vi "WSVCAP SHL Host TL Tester.vi"() -> ()   [LabVIEW 2012]
uses:
  Type Defs/WSVCAP SHL DUT Number Enum.ctl
  <vilib>/userdefined/High Color/nirio_resource_hc.ctl
  Type Defs/WSVCAP SHL Tester System Cluster.ctl
  Type Defs/WSVCAP SHL I2C DUT Mask Mode Enum.ctl
panel:
  in  "Mode":enum32{"C1", "C2", "C3", "All", "Single"}(radio)
  in  "RFFE Slave Address":u8=144 caption="Slave Address" format="0x%02x"
  in  "RFFE Mode":enum32{"Write/Read", "Cycle"}(tab)
  in  "Read Data DUT":string caption="Read Data Out"
  in  "Read DUT":bool
  in  "Enable DUT":bool
  in  "Disable DUT":bool
  in  "Write DUT":bool
  in  "Write Data DUT":string caption="Write Data Out"
  out "Read Data DUT":string caption="Data In"
  out "Cycle Count":u64=2 min=1 max=4 step=1 format="%#.4p"
  in  "Number of Commands":u32=2 min=1 max=4 step=1
  in  "Post Command Delay":dbl[](array[numeric])=[5e-06, 5e-06] min=0.0 max=0.5 format="%#.0p s"
  in  "Command":string[](array[string])=["4200000000", "421F7F1F7F"]
  in  "Start RFFE Cycle":bool
  in  "Stop RFFE Cycle":bool
  out "Activity Log":string
  out "Simulate FPGA":bool
  out "Online":bool
  out "FPGA Resource":T1
  out "Status":string
  out "Busy":bool
  in  "I2C Bytes to Read":u8=1 caption="Bytes" min=1 max=4 step=1
  in  "Device":enum32{"C1", "C2", "C3"}(radio)
  in  "Exit":bool
  out "Read Data I2C":u8[](array[numeric]) caption="Data In" format="0x%02x"
  in  "Read Reg I2C":u8 caption="Register" format="0x%02x"
  in  "Read I2C":bool
  in  "DUT":T2
  in  "Write Data I2C":u8 caption="Data Out" format="0x%02x"
  in  "Write Reg I2C":u8=144 caption="Register" format="0x%02x"
  in  "I2C Init":bool
  in  "Init Data":u8[](array[numeric])=[164, 160, 14, 33] caption="Data Out" format="0x%02x"
  in  "Init Reg":u8[](array[numeric])=[191, 7, 9, 10] caption="Register" format="0x%02x"
  in  "Write I2C":bool
  in  "Monitor":bool
  in  "I2C Slave Address":u8=144 caption="Slave Address" format="0x%02x"
  out "AD7747 Values":string[][](table)
  in  "RFFE Clock Rate (Hz)":dbl=1000000.0 caption="Clock Rate" format="%.1p Hz"
  in  "I2C Clock Rate (Hz)":dbl=100000.0 caption="Clock Rate" format="%.0p Hz"
  in  "Error":errorcluster
  # "WS1050 Tester"
  # "AD7747 (I2C)"
  # "DUT (RFFE)"
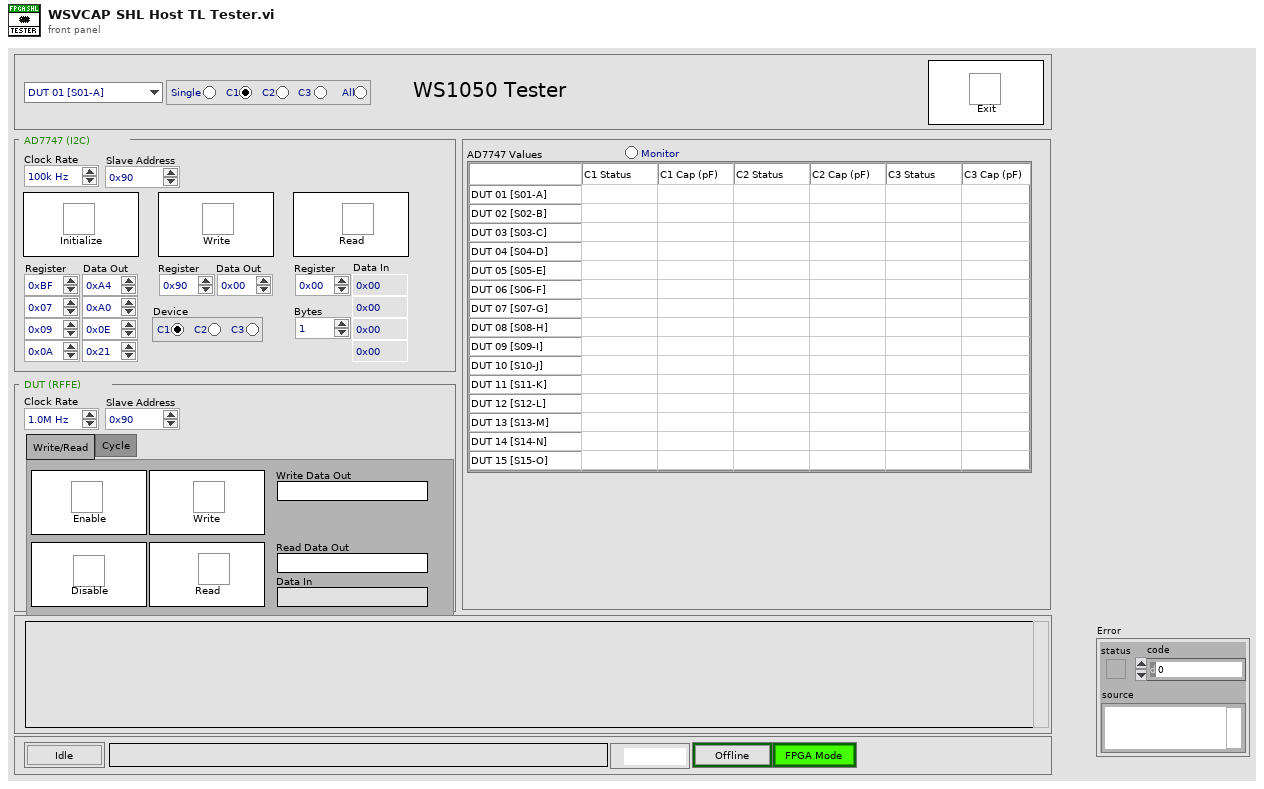
[diagram p1: front panel]
types:
  T1 = typedef "nirio_resource_hc.ctl" = tag
  T2 = typedef "WSVCAP SHL DUT Number Enum.ctl" = enum16{"DUT 01 [S01-A]", "DUT 02 [S02-B]", "DUT 03 [S03-C]", "DUT 04 [S04-D]", "DUT 05 [S05-E]", "DUT 06 [S06-F]", "DUT 07 [S07-G]", "DUT 08 [S08-H]", "DUT 09 [S09-I]", "DUT 10 [S10-J]", "DUT 11 [S11-K]", "DUT 12 [S12-L]", "DUT 13 [S13-M]", "DUT 14 [S14-N]", "DUT 15 [S15-O]", "DUT 16 [S16-P]"}
  T3 = typedef "WSVCAP SHL Tester System Cluster.ctl" = cluster{"I2C Monitor":bool, "SPI Cyle":bool, "SPI Mode":enum32{"Write/Read", "Cycle"}, "RFFE Cyle":bool, "RFFE Mode":enum32{"Write/Read", "Cycle"}}
  T4 = enum8{"Enabled", "Disabled", "Disabled and Grayed Out"}
  T5 = typedef "WSVCAP SHL I2C DUT Mask Mode Enum.ctl" = enum16{"Custom", "C1", "C2", "C3", "All"}
  T6 = typedef "WSVCAP SHL Core System Cluster.ctl" = cluster{"Settings":T7, "FPGA Resource":tag, "Online":bool, "I2C Wait Ticks":u32, "SPI Wait Ticks":u32, "RFFE Wait Ticks":u32}
  T7 = typedef "WSVCAP SHL I2C Settings Cluster.ctl" = cluster{"FPGA Resource Name":string, "I2C Slave Address":u8, "I2C Clock Rate (Hz)":dbl, "SPI Clock Rate (Hz)":dbl, "RFFE Slave Address":u8, "RFFE Clock Rate (Hz)":dbl, "Simulate FPGA":bool}
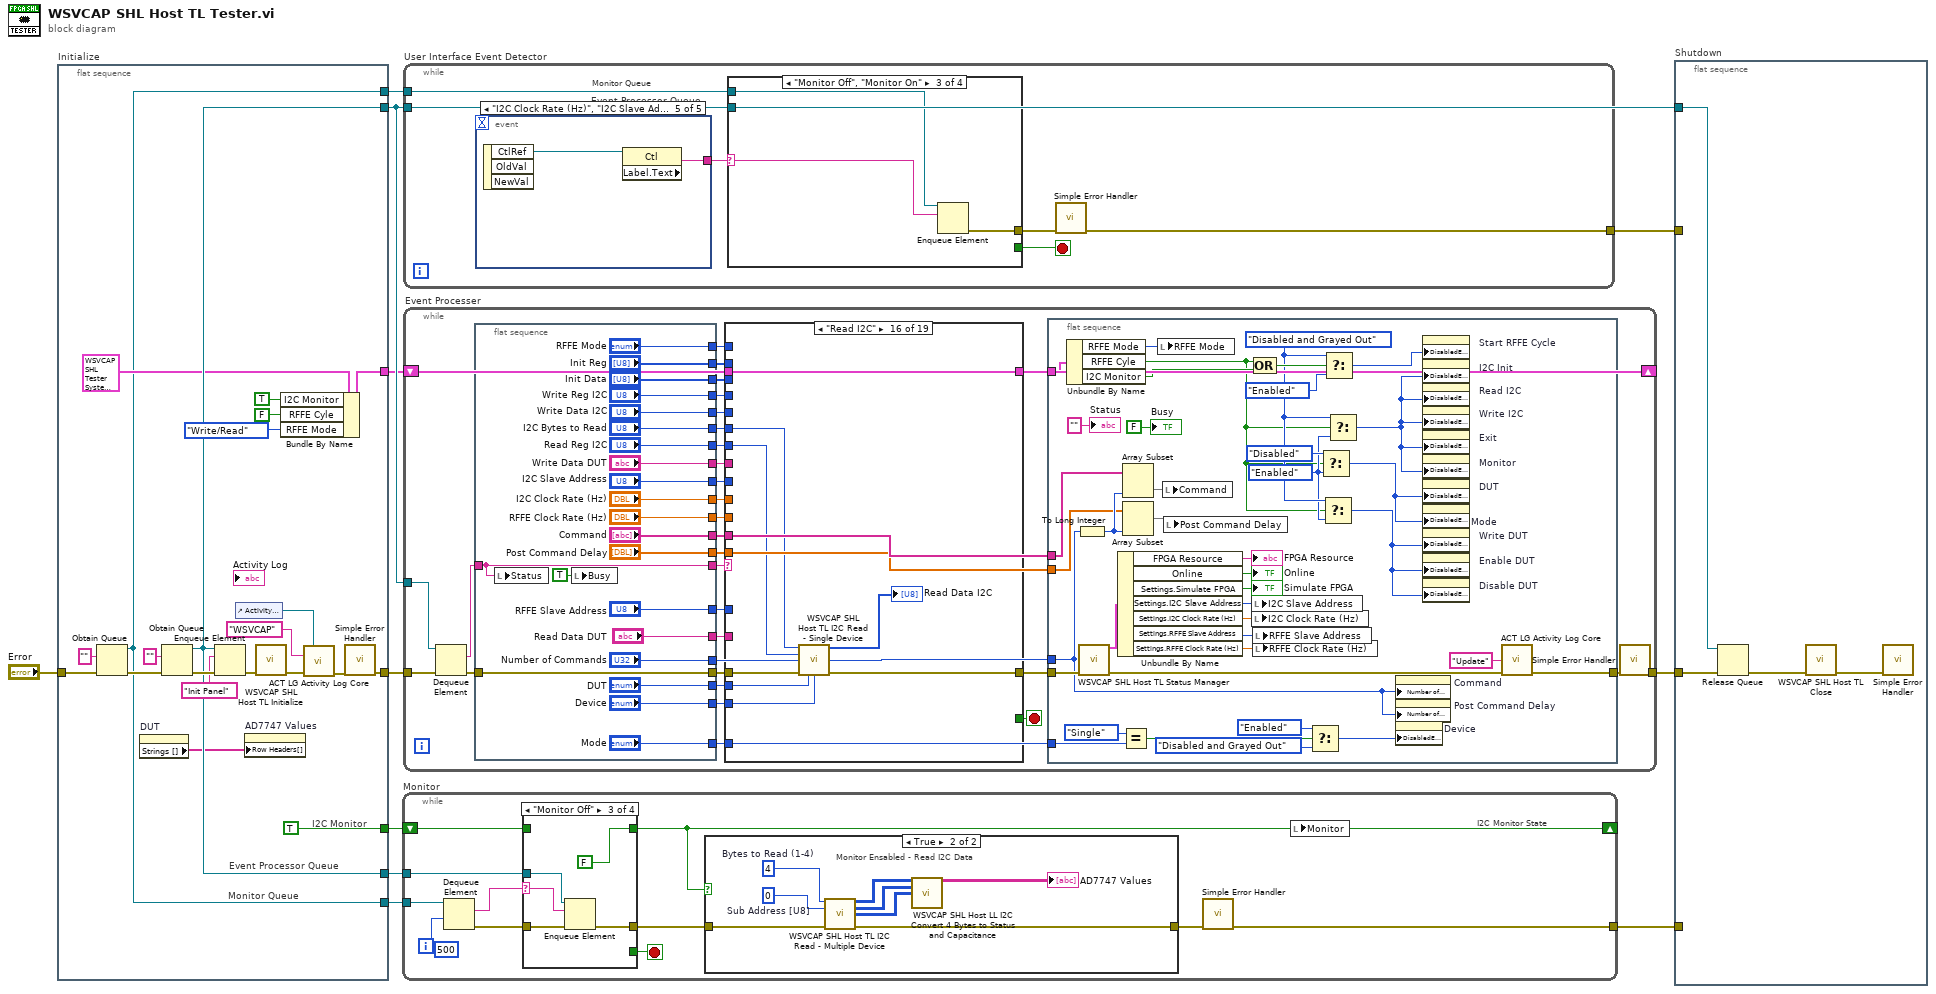
[diagram p0: block diagram]
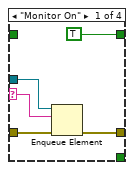
[diagram p2: hidden frame]
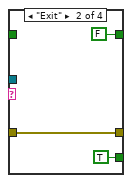
[diagram p3: hidden frame]
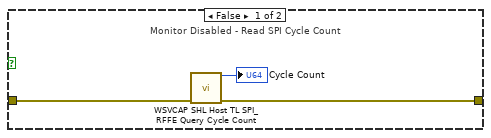
[diagram p5: hidden frame]
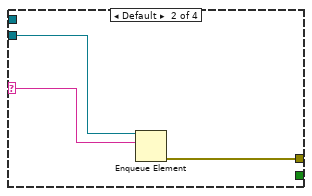
[diagram p7: hidden frame]
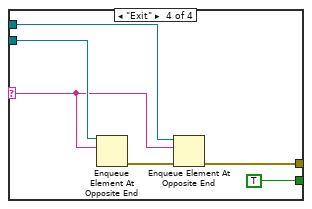
[diagram p8: hidden frame]
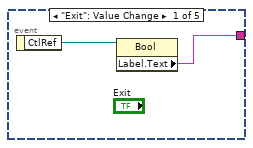
[diagram p9: hidden frame]
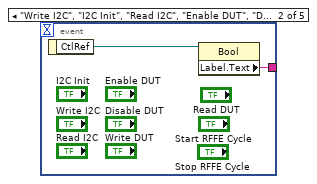
[diagram p10: hidden frame]
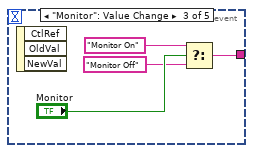
[diagram p11: hidden frame]
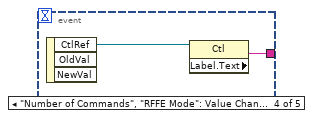
[diagram p12: hidden frame]
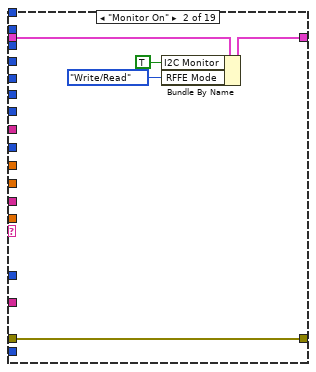
[diagram p14: hidden frame]
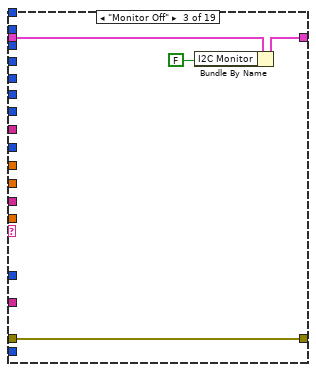
[diagram p15: hidden frame]
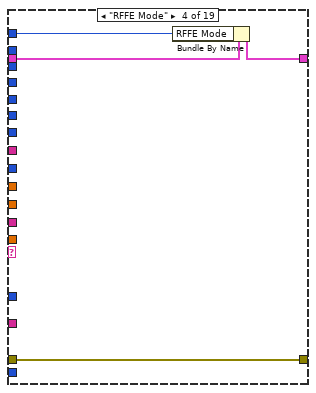
[diagram p16: hidden frame]
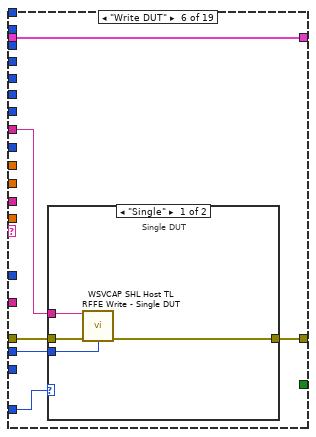
[diagram p18: hidden frame]
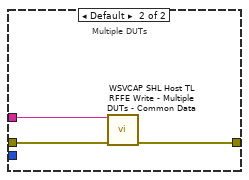
[diagram p19: hidden frame]
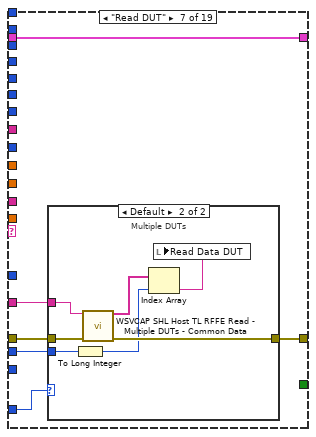
[diagram p20: hidden frame]
diagram:
  n1 = flat-sequence "Initialize" {
    tunnel: "Error" -> [w21]
    tunnel: [w19] -> w10
    tunnel: [TRUE ("Monitor")] -> w1
    tunnel: [w26] -> w6
    tunnel: [w17] -> w5
    tunnel: [w14] -> w4
    tunnel: [w19] -> w3
    tunnel: [w14] -> w2
    frame #0 {
      # "I2C Monitor"
      # "Monitor Queue"
      # "Event Processor Queue"
      n2 = Obtain Queue(element data type="" ("name (unnamed)"), error in (no error)=w21) -> (queue out=w14:refnum<queue>, error out=w20:errorcluster)  [unwired: 3 in, 1 out]
      n3 = property on="DUT" class="Enum (strict)"() -> ("Strings []"=w12:string[])  [unwired: 2 in, 2 out]
      n4 = Obtain Queue(element data type="" ("name (unnamed)"), error in (no error)=w20) -> (queue out=w19:refnum<queue>, error out=w31:errorcluster)  [unwired: 3 in, 1 out]
      n5 = Enqueue Element(queue=w19, element="Init Panel" ("name (unnamed)"), error in (no error)=w31) -> (error out=w30:errorcluster)  [unwired: 1 in, 2 out]
      n6 = control-ref of="Activity Log"() -> (w25:refnum<vi>)
      n7 = property on="AD7747 Values" class="Tbl (strict)"("Row Headers[]"=w12) -> ()  [unwired: 2 in, 2 out]
      n8 = call "WSVCAP SHL Host TL Initialize.vi"("error in"=w30) -> ("error out"=w28:errorcluster)  [unwired: 14 in]
      n9 = Bundle By Name(cluster=T3 {"I2C Monitor"=TRUE, "SPI Cyle"=TRUE, "SPI Mode"=enum."Write/Read", "RFFE Cyle"=FALSE, "RFFE Mode"=enum."Write/Read"}, "I2C Monitor"=TRUE, "RFFE Cyle"=FALSE ("I2C Monitor"), "RFFE Mode"=enum32{"Write/Read", "Cycle"}."Write/Read" ("SPI Mode")) -> (w17:T3)
      n10 = call "ACT LG Activity Log Core.vi"("Display Ref"=w25, "Source"="WSVCAP", "Error In (no error)"=w28) -> ("Error Out"=w27:errorcluster)  [unwired: 11 in, 1 out]
      n11 = call <vilib>:"Simple Error Handler.vi"("error in (no error)"=w27) -> ("error out"=w26:errorcluster)  [unwired: 4 in, 4 out]
    }
  }
  n12 = while "Monitor" {
    tunnel: [w34] -> w7
    shift-right: [w33] -> _
    shift-left: w1 -> [w40]
    tunnel: w4 -> [w38]
    tunnel: w3 -> [w37]
    stop <- w35 stop-if-true
    # "I2C Monitor State"
    n13 = Dequeue Element(queue=w38, timeout in ms (-1)=500 ("Wait Time (500ms)")) -> (element=w41:string, error out=w39:errorcluster)  [unwired: 1 in, 2 out]
    n14 = case shown="\"Monitor Off\"" w41 {
      selector: w41 -> [w45 _ w53 _]
      tunnel: [TRUE FALSE FALSE w58] -> w33
      tunnel: w40 -> [_ _ _ w58]
      tunnel: w39 -> [w47 w50 w55 w57]
      tunnel: [w46 w50 w54 w57] -> w36
      tunnel: w37 -> [w44 _ w52 _]
      tunnel: [_ TRUE _ _] -> w35
      frame "Monitor On" {
        n15 = Enqueue Element(queue=w44, element=w45, error in (no error)=w47) -> (error out=w46:errorcluster)  [unwired: 1 in, 2 out]
      }
      frame "Exit" {
      }
      frame "Monitor Off" {
        n16 = Enqueue Element(queue=w52, element=w53, error in (no error)=w55) -> (error out=w54:errorcluster)  [unwired: 1 in, 2 out]
      }
      frame Default {
      }
    }
    n17 = case shown="True" w33 {
      tunnel: [w59 w63] -> w43
      tunnel: w36 -> [w60 w64]
      frame False {
        # "Monitor Disabled - Read SPI Cycle Count"
        n18 = call "WSVCAP SHL Host TL SPI_RFFE Query Cycle Count.vi"("error in"=w60) -> ("Cycle Count"=→"Cycle Count":u64, "error out"=w59:errorcluster)  [unwired: 13 in]
      }
      frame True {
        w68 = u8 4  # Bytes to Read (1-4)
        w69 = u8 0  # Sub Address [U8]
        # "Monitor Ensabled - Read I2C Data"
        n19 = call "WSVCAP SHL Host TL I2C Read - Multiple Device.vi"("Bytes to Read (1-4)"=w68, "Sub Address [U8]"=w69, "error in"=w64) -> ("C1:1-16 Read Data [U8]"=w67:u8[][], "C2:1-16 Read Data [U8]"=w66:u8[][], "C3:1-16 Read Data [U8]"=w62:u8[][], "error out"=w63:errorcluster)  [unwired: 9 in]
        n20 = call "WSVCAP SHL Host LL I2C Convert 4 Bytes to Status and Capacitance.vi"("C1:1-16 Read Data [U8]"=w67, "C2_1-16 Read Data [U8]"=w66, "C3_1-16 Read Data [U8]"=w62) -> ("AD7747 Values"=→"AD7747 Values":string[][])  [unwired: 12 in]
      }
    }
    n21 = call <vilib>:"Simple Error Handler.vi"("error in (no error)"=w43) -> ("error out"=w34:errorcluster)  [unwired: 4 in, 4 out]
    n22 = local write "Monitor"(w33) -> ()
  }
  n23 = while "User Interface Event Detector" {
    tunnel: w10 -> [w74]
    tunnel: [w71] -> w8
    tunnel: w2 -> [w70]
    stop <- w72 stop-if-true
    # "Monitor Queue"
    # "Event Processor Queue"
    n24 = event shown="[4] \"I2C Clock Rate (Hz)\", \"I2C Slave Address\", \"RFFE Clock Rate (Hz)\", \"RFFE Slave Address\", \"Mode\": Value Change" {
      selector: _ -> [_ _ _ _ _]
      dyn-events: _ -> [_ _ _ _ _]
      timeout: _ -> [_ _ _ _ _]
      tunnel: [w88 w91 w92 w97 w99] -> w75
      event "Exit": Value Change {
        n25 = event-data() -> ("CtlRef"=w89:refnum<vi>)  [unwired: 1 in]
        n26 = property class="Bool"(reference=w89) -> ("Label.Text"=w88:string)  [unwired: 1 in, 2 out]
      }
      event "Write I2C", "I2C Init", "Read I2C", "Enable DUT", "Disable DUT", "Write DUT", "Start RFFE Cycle", "Stop RFFE Cycle", "Read DUT": Value Change {
        n27 = event-data() -> ("CtlRef"=w90:refnum<vi>)  [unwired: 1 in]
        n28 = property class="Bool"(reference=w90) -> ("Label.Text"=w91:string)  [unwired: 1 in, 2 out]
      }
      event "Monitor": Value Change {
        n29 = event-data() -> ()  [unwired: 1 in, 3 out]
        n30 = Select(t="Monitor On" ("Label.Text"), s="Monitor", f="Monitor Off" ("Label.Text")) -> (s? t:f=w92:string)
      }
      event "Number of Commands", "RFFE Mode": Value Change {
        n31 = event-data() -> ("CtlRef"=w96:refnum<vi>)  [unwired: 1 in, 2 out]
        n32 = property class="Ctl"(reference=w96) -> ("Label.Text"=w97:string)  [unwired: 1 in, 2 out]
      }
      event "I2C Clock Rate (Hz)", "I2C Slave Address", "RFFE Clock Rate (Hz)", "RFFE Slave Address", "Mode": Value Change {
        n33 = event-data() -> ("CtlRef"=w98:refnum<vi>)  [unwired: 1 in, 2 out]
        n34 = property class="Ctl"(reference=w98) -> ("Label.Text"=w99:string)  [unwired: 1 in, 2 out]
      }
    }
    n35 = case shown="\"Monitor Off\", \"Monitor On\"" w75 {
      selector: w75 -> [_ w78 w81 w82]
      tunnel: w74 -> [_ w77 _ w87]
      tunnel: [_ w76 w80 w84] -> w73
      tunnel: [_ _ _ TRUE] -> w72
      tunnel: w70 -> [_ _ w79 w83]
      frame "" {
      }
      frame Default {
        n36 = Enqueue Element(queue=w77, element=w78) -> (error out=w76:errorcluster)  [unwired: 2 in, 2 out]
      }
      frame "Monitor Off", "Monitor On" {
        n37 = Enqueue Element(queue=w79, element=w81) -> (error out=w80:errorcluster)  [unwired: 2 in, 2 out]
      }
      frame "Exit" {
        n38 = Enqueue Element At Opposite End(queue=w87, element=w82) -> (error out=w85:errorcluster)  [unwired: 2 in, 2 out]
        n39 = Enqueue Element At Opposite End(queue=w83, element=w82, error in (no error)=w85) -> (error out=w84:errorcluster)  [unwired: 1 in, 2 out]
      }
    }
    n40 = call <vilib>:"Simple Error Handler.vi"("error in (no error)"=w73) -> ("error out"=w71:errorcluster)  [unwired: 4 in, 4 out]
  }
  n41 = while "Event Processer" {
    tunnel: w10 -> [w130]
    tunnel: [w128] -> w9
    tunnel: w6 -> [w109]
    shift-right: [w103] -> _
    shift-left: w5 -> [w104]
    stop <- w129 stop-if-true
    n42 = Dequeue Element(queue=w130, error in (no error)=w109) -> (element=w126:string, error out=w124:errorcluster)  [unwired: 1 in, 2 out]
    n43 = flat-sequence {
      tunnel: ["I2C Clock Rate (Hz)"] -> w127
      tunnel: [w177] -> w125
      tunnel: w126 -> [w177]
      tunnel: [w190] -> w123
      tunnel: w124 -> [w190]
      tunnel: ["I2C Bytes to Read"] -> w122
      tunnel: ["I2C Slave Address"] -> w121
      tunnel: ["RFFE Clock Rate (Hz)"] -> w120
      tunnel: ["DUT"] -> w117
      tunnel: ["Init Data"] -> w116
      tunnel: ["Init Reg"] -> w115
      tunnel: ["Write Reg I2C"] -> w114
      tunnel: ["Write Data I2C"] -> w113
      tunnel: ["Read Reg I2C"] -> w112
      tunnel: ["Write Data DUT"] -> w111
      tunnel: ["Mode"] -> w100
      tunnel: ["Device"] -> w110
      tunnel: ["RFFE Mode"] -> w108
      tunnel: ["Command"] -> w106
      tunnel: ["Post Command Delay"] -> w105
      tunnel: ["Number of Commands"] -> w107
      tunnel: ["RFFE Slave Address"] -> w102
      tunnel: ["Read Data DUT"] -> w101
      frame #0 {
        n44 = local write "Status"(w177) -> ()
        n45 = local write "Busy"(TRUE ("Busy")) -> ()
      }
    }
    n46 = case shown="\"Read I2C\"" w125 {
      selector: w125 -> [_ _ _ _ _ _ _ _ _ _ _ _ w305 _ _ _ _ _ _]
      tunnel: w123 -> [w193 w198 w202 w206 w208 w214 w227 w245 w261 w279 w293 w298 w309 w324 w346 w375 w377 w383 w388]
      tunnel: [w193 w198 w202 w206 w208 w213 w226 w244 w260 w278 w292 w297 w308 w323 w345 w369 w377 w380 w386] -> w119
      tunnel: [_ _ _ _ _ _ _ _ _ _ _ _ _ _ _ _ TRUE _ _] -> w129
      tunnel: w127 -> [_ _ _ _ _ _ _ _ _ _ _ _ _ _ _ _ _ w382 _]
      tunnel: w122 -> [_ _ _ _ _ _ _ _ _ _ _ _ _ _ _ w371 _ _ _]
      tunnel: w121 -> [_ _ _ _ _ _ _ _ _ _ _ _ _ _ _ _ _ w381 _]
      tunnel: w120 -> [_ _ _ _ _ _ _ _ _ _ _ _ _ _ _ _ _ _ w387]
      tunnel: w117 -> [_ _ _ _ _ w211 w224 w242 w258 w276 _ _ w306 w321 w343 w374 _ _ _]
      tunnel: w116 -> [_ _ _ _ _ _ _ _ _ _ _ _ _ _ w340 _ _ _ _]
      tunnel: w115 -> [_ _ _ _ _ _ _ _ _ _ _ _ _ _ w341 _ _ _ _]
      tunnel: w114 -> [_ _ _ _ _ _ _ _ _ _ _ _ _ w319 _ _ _ _ _]
      tunnel: w113 -> [_ _ _ _ _ _ _ _ _ _ _ _ _ w318 _ _ _ _ _]
      tunnel: w112 -> [_ _ _ _ _ _ _ _ _ _ _ _ _ _ _ w372 _ _ _]
      tunnel: w111 -> [_ _ _ _ _ w210 _ w241 _ _ _ _ _ _ _ _ _ _ _]
      tunnel: w100 -> [_ _ _ _ _ w212 w225 w243 w259 w277 _ _ w307 w322 w344 _ _ _ _]
      tunnel: w110 -> [_ _ _ _ _ _ _ _ _ _ _ _ _ w320 w342 w373 _ _ _]
      tunnel: w108 -> [_ _ _ w203 _ _ _ _ _ _ _ _ _ _ _ _ _ _ _]
      tunnel: w106 -> [_ _ _ _ _ _ _ _ w257 w275 _ _ _ _ _ _ _ _ _]
      tunnel: w105 -> [_ _ _ _ _ _ _ _ w256 w274 _ _ _ _ _ _ _ _ _]
      tunnel: [w192 w196 w200 w204 w207 w209 w223 w240 w254 w272 w289 w294 w299 w317 w339 w368 w376 w379 w385] -> w103
      tunnel: w104 -> [w192 w197 w201 w205 w207 w209 w223 w240 w255 w273 w290 w295 w299 w317 w339 w368 w376 w379 w385]
      tunnel: w102 -> [_ _ _ _ _ _ _ _ _ _ _ _ _ _ _ _ _ _ w384]
      tunnel: w101 -> [_ _ _ _ _ _ w222 _ _ _ _ _ _ _ _ _ _ _ _]
      frame Default {
      }
      frame "Monitor On" {
        n47 = Bundle By Name(cluster=w197, "I2C Monitor"=TRUE, "RFFE Mode"=enum32{"Write/Read", "Cycle"}."Write/Read" ("SPI Mode")) -> (w196:T3)
      }
      frame "Monitor Off" {
        n48 = Bundle By Name(cluster=w201, "I2C Monitor"=FALSE) -> (w200:T3)
      }
      frame "RFFE Mode" {
        n49 = Bundle By Name(cluster=w205, "RFFE Mode"=w203) -> (w204:T3)
      }
      frame "Number of Commands" {
      }
      frame "Write DUT" {
        n50 = case shown="\"Single\"" w212 {
          tunnel: w214 -> [w218 w221]
          tunnel: [w215 w220] -> w213
          tunnel: w211 -> [w216 _]
          tunnel: w210 -> [w217 w219]
          frame "Single" {
            # "Single DUT"
            n51 = call "WSVCAP SHL Host TL RFFE Write - Single DUT.vi"("Data Out"=w217, "error in"=w218, "DUT"=w216) -> ("error out"=w215:errorcluster)  [unwired: 12 in]
          }
          frame Default {
            # "Multiple DUTs"
            n52 = call "WSVCAP SHL Host TL RFFE Write - Multiple DUTs - Common Data.vi"("Data Out"=w219, "error in"=w221) -> ("error out"=w220:errorcluster)  [unwired: 13 in]
          }
        }
      }
      frame "Read DUT" {
        n53 = case shown="Default" w225 {
          tunnel: w227 -> [w232 w239]
          tunnel: [w230 w238] -> w226
          tunnel: w224 -> [w231 w235]
          tunnel: w222 -> [w228 w237]
          frame "Single" {
            # "Single DUT"
            n54 = call "WSVCAP SHL Host TL RFFE Read - Single DUT.vi"("Data Out"=w228, "error in"=w232, "DUT"=w231) -> ("Data In"=→"Read Data DUT":string, "error out"=w230:errorcluster)  [unwired: 11 in]
          }
          frame Default {
            # "Multiple DUTs"
            n55 = To Long Integer(number=w235) -> (32bit integer=w234:i32)
            n56 = call "WSVCAP SHL Host TL RFFE Read - Multiple DUTs - Common Data.vi"("Data Out"=w237, "error in"=w239) -> ("RFFE Data In"=w236:string[], "error out"=w238:errorcluster)  [unwired: 12 in]
            n57 = Index Array(array=w236, index=w234) -> (element=w233:string)
            n58 = local write "Read Data DUT"(w233) -> ()
          }
        }
      }
      frame "Write/Read DUT" {
        n59 = case shown="\"C2\"" w243 {
          tunnel: w245 -> [w249 w252]
          tunnel: [w247 w251] -> w244
          tunnel: w242 -> [w248 _]
          tunnel: w241 -> [w246 w250]
          frame "C1", Default {
            # "Single DUT"
            n60 = call "WSVCAP SHL Host TL SPI Write_Read - Single DUT.vi"("Data Out"=w246, "error in"=w249, "DUT"=w248) -> ("error out"=w247:errorcluster)  [unwired: 11 in, 1 out]
          }
          frame "C2" {
            # "Multiple DUTs"
            n61 = call "WSVCAP SHL Host TL SPI Write_Read - Multiple DUTs - Common Data.vi"("Data Out"=w250, "error in"=w252) -> ("error out"=w251:errorcluster)  [unwired: 12 in, 1 out]
          }
        }
      }
      frame "Start SPI Cycle" {
        n62 = case shown="\"C2\"" w259 {
          tunnel: w261 -> [w266 w270]
          tunnel: [w265 w269] -> w260
          tunnel: w258 -> [w264 _]
          tunnel: w257 -> [w263 w268]
          tunnel: w256 -> [w262 w267]
          frame "C1", Default {
            # "Single DUT"
            n63 = call "WSVCAP SHL Host TL SPI Write Cycle - Single DUT.vi"("Data Out (Cycle Commands)"=w263, "Post Command Delay"=w262, "error in"=w266, "DUT"=w264) -> ("error out"=w265:errorcluster)  [unwired: 11 in]
          }
          frame "C2" {
            # "Multiple DUTs"
            n64 = call "WSVCAP SHL Host TL SPI Write Cycle - Multiple DUTs - Common Data.vi"("Data Out (Cycle Commands)"=w268, "Post Command Delay"=w267, "error in"=w270) -> ("error out"=w269:errorcluster)  [unwired: 12 in]
          }
        }
        n65 = Bundle By Name(cluster=w255, "SPI Cyle"=TRUE) -> (w254:T3)
      }
      frame "Start RFFE Cycle" {
        n66 = case shown="\"C2\"" w277 {
          tunnel: w279 -> [w284 w288]
          tunnel: [w283 w287] -> w278
          tunnel: w276 -> [w282 _]
          tunnel: w275 -> [w281 w286]
          tunnel: w274 -> [w280 w285]
          frame "C1", Default {
            # "Single DUT"
            n67 = call "WSVCAP SHL Host TL RFFE Write Cycle - Single DUT.vi"("Data Out (Cycle Commands)"=w281, "Post Command Delay"=w280, "error in"=w284, "DUT"=w282) -> ("error out"=w283:errorcluster)  [unwired: 11 in]
          }
          frame "C2" {
            # "Multiple DUTs"
            n68 = call "WSVCAP SHL Host TL RFFE Write Cycle - Multiple DUTs - Common Data.vi"("Data Out (Cycle Commands)"=w286, "Post Command Delay"=w285, "error in"=w288) -> ("error out"=w287:errorcluster)  [unwired: 12 in]
          }
        }
        n69 = Bundle By Name(cluster=w273, "RFFE Cyle"=TRUE ("SPI Cyle")) -> (w272:T3)
      }
      frame "Stop RFFE Cycle" {
        n70 = call "WSVCAP SHL Host TL RFFE Stop Write Cycle.vi"("error in"=w293) -> ("error out"=w292:errorcluster)  [unwired: 14 in]
        n71 = Bundle By Name(cluster=w290, "RFFE Cyle"=FALSE ("SPI Cyle")) -> (w289:T3)
      }
      frame "Stop SPI Cycle" {
        n72 = call "WSVCAP SHL Host TL SPI Stop Write Cycle.vi"("error in"=w298) -> ("error out"=w297:errorcluster)  [unwired: 14 in]
        n73 = Bundle By Name(cluster=w295, "SPI Cyle"=FALSE) -> (w294:T3)
      }
      frame "Disable DUT", "Enable DUT" {
        n74 = Equal?(x="Enable DUT", y=w305) -> (x = y?=w303:bool)
        n75 = Select(t="0040" ("Data Out"), s=w303, f="0000" ("Data Out")) -> (s? t:f=w302:string)
        n76 = case shown="\"C2\"" w307 {
          tunnel: w309 -> [w313 w316]
          tunnel: [w312 w315] -> w308
          tunnel: w306 -> [w311 _]
          tunnel: w302 -> [w310 w314]
          frame "C1", Default {
            # "Single DUT"
            n77 = call "WSVCAP SHL Host TL RFFE Write - Single DUT.vi"("Data Out"=w310, "error in"=w313, "DUT"=w311) -> ("error out"=w312:errorcluster)  [unwired: 12 in]
          }
          frame "C2" {
            # "Multiple DUTs"
            n78 = call "WSVCAP SHL Host TL RFFE Write - Multiple DUTs - Common Data.vi"("Data Out"=w314, "error in"=w316) -> ("error out"=w315:errorcluster)  [unwired: 13 in]
          }
        }
      }
      frame "Write I2C" {
        n79 = case shown="Default" w322 {
          selector: w322 -> [_ w334]
          tunnel: w324 -> [w330 w338]
          tunnel: [w329 w337] -> w323
          tunnel: w321 -> [w327 _]
          tunnel: w319 -> [w326 w336]
          tunnel: w320 -> [w328 _]
          tunnel: w318 -> [w325 w335]
          frame "Single" {
            # "Single DUT"
            n80 = call "WSVCAP SHL Host TL I2C Write - Single Device.vi"("Sub Address [U8]"=w326, "Data Out [U8]"=w325, "error in"=w330, "DUT"=w327, "Device"=w328) -> ("error out"=w329:errorcluster)  [unwired: 10 in]
          }
          frame Default {
            # "Multiple DUTs"
            n81 = Format Into String(w334) -> (resulting string=w333:string)  [unwired: 3 in, 1 out]
            n82 = Scan From String(input string=w333, default 1=WSVCAP_SHL_I2C_DUT_Mask_Mode_Enum."All" ("DUT Mask Mode (All)")) -> (output 1=w331:T5)  [unwired: 3 in, 3 out]
            n83 = call "WSVCAP SHL Host TL I2C Write - Multiple Device - Common Data.vi"("Sub Address"=w336, "Data Out [U8]"=w335, "error in"=w338, "DUT Mask Mode (All)"=w331) -> ("error out"=w337:errorcluster)  [unwired: 11 in]
          }
        }
      }
      frame "I2C Init" {
        n84 = for {
          tunnel: w344 -> [w351]
          tunnel: w343 -> [w350]
          tunnel: w342 -> [w349]
          tunnel: w341 -> [w348] mode=indexing
          tunnel: w340 -> [w347] mode=indexing
          shift-right: [w352] -> w345
          shift-left: w346 -> [w353]
          n85 = case shown="Default" w351 {
            selector: w351 -> [_ w361]
            tunnel: w353 -> [w359 w367]
            tunnel: [w358 w366] -> w352
            tunnel: w350 -> [w356 _]
            tunnel: w349 -> [w357 _]
            tunnel: w348 -> [w355 w365]
            tunnel: w347 -> [w354 w364]
            frame "Single" {
              # "Single DUT"
              n86 = call "WSVCAP SHL Host TL I2C Write - Single Device.vi"("Sub Address [U8]"=w355, "Data Out [U8]"=w354, "error in"=w359, "DUT"=w356, "Device"=w357) -> ("error out"=w358:errorcluster)  [unwired: 10 in]
            }
            frame Default {
              # "Multiple DUTs"
              n87 = Format Into String(w361) -> (resulting string=w363:string)  [unwired: 3 in, 1 out]
              n88 = Scan From String(input string=w363, default 1=WSVCAP_SHL_I2C_DUT_Mask_Mode_Enum."All" ("DUT Mask Mode (All)")) -> (output 1=w360:T5)  [unwired: 3 in, 3 out]
              n89 = call "WSVCAP SHL Host TL I2C Write - Multiple Device - Common Data.vi"("Sub Address"=w365, "Data Out [U8]"=w364, "error in"=w367, "DUT Mask Mode (All)"=w360) -> ("error out"=w366:errorcluster)  [unwired: 11 in]
            }
          }
        }
      }
      frame "Read I2C" {
        n90 = call "WSVCAP SHL Host TL I2C Read - Single Device.vi"("Bytes to Read (1-4)"=w371, "Sub Address [U8]"=w372, "error in"=w375, "DUT"=w374, "Device"=w373) -> ("Device Data"=→"Read Data I2C":u8[], "error out"=w369:errorcluster)  [unwired: 9 in]
      }
      frame "Exit" {
      }
      frame "I2C Clock Rate (Hz)", "I2C Slave Address" {
        n91 = call "WSVCAP SHL Host TL I2C Configure.vi"("I2C_Slave Address"=w381, "Clock Rate (Hz)"=w382, "error in"=w383) -> ("error out"=w380:errorcluster)  [unwired: 11 in, 1 out]
      }
      frame "RFFE Clock Rate (Hz)", "RFFE Slave Address" {
        n92 = call "WSVCAP SHL Host TL RFFE Configure.vi"("RFFE Slave Address"=w384, "Clock Rate (Hz)"=w387, "error in"=w388) -> ("error out"=w386:errorcluster)  [unwired: 11 in, 1 out]
      }
    }
    n93 = flat-sequence {
      tunnel: [w157] -> w118
      tunnel: w119 -> [w167]
      tunnel: w107 -> [w156]
      tunnel: w106 -> [w154]
      tunnel: w105 -> [w152]
      tunnel: w103 -> [w150]
      tunnel: w100 -> [w136]
      frame #0 {
        w143 = T4."Enabled" ("Disabled")
        w144 = T4."Disabled and Grayed Out" ("Disabled")
        n94 = Unbundle By Name(w150) -> ("RFFE Mode"=w149:enum32{"Write/Read", "Cycle"}, "RFFE Cyle"=w141:bool, "I2C Monitor"=w148:bool)
        n95 = To Long Integer(number=w156) -> (32bit integer=w155:i32)
        n96 = call "WSVCAP SHL Host TL Status Manager.vi"("error in"=w167) -> ("System Out"=w166:T6, "error out"=w159:errorcluster)  [unwired: 13 in]
        n97 = Unbundle By Name(w166) -> ("FPGA Resource"=→"FPGA Resource":tag, "Online"=→"Online":bool, "Settings.Simulate FPGA"=→"Simulate FPGA":bool, "Settings.I2C Slave Address"=w165:u8, "Settings.I2C Clock Rate (Hz)"=w164:dbl, "Settings.RFFE Slave Address"=w138:u8, "Settings.RFFE Clock Rate (Hz)"=w163:dbl)
        n98 = Equal?(x=enum32{"C1", "C2", "C3", "All", "Single"}."Single" ("Mode"), y=w136) -> (x = y?=w132:bool)
        n99 = Array Subset(array=w154, length=w155) -> (w153:string[])  [unwired: 1 in]
        n100 = Array Subset(array=w152, length=w155) -> (w151:dbl[])  [unwired: 1 in]
        n101 = local write "RFFE Mode"(w149) -> ()
        n102 = local write "Command"(w153) -> ()
        n103 = local write "Post Command Delay"(w151) -> ()
        n104 = local write "I2C Slave Address"(w165) -> ()
        n105 = local write "I2C Clock Rate (Hz)"(w164) -> ()
        n106 = local write "RFFE Slave Address"(w138) -> ()
        n107 = local write "RFFE Clock Rate (Hz)"(w163) -> ()
        n108 = Compound Arithmetic op=OR(w141, w148) -> (w145:bool)
        n109 = Select(t=T4."Enabled" ("Disabled"), s=w132, f=T4."Disabled and Grayed Out" ("Disabled")) -> (s? t:f=w131:T4)
        n110 = Select(t=T4."Disabled" ("Disabled"), s=w141, f=w143) -> (s? t:f=w137:T4)
        n111 = Select(t=w144, s=w141, f=w143) -> (s? t:f=w142:T4)
        n112 = Select(t=w144, s=w145, f=T4."Enabled" ("Disabled")) -> (s? t:f=w140:T4)
        n113 = Select(t=w144, s=w141, f=w143) -> (s? t:f=w139:T4)
        n114 = property on="Command" class="Arr (strict)"("Number of Rows"=w156) -> ()  [unwired: 2 in, 2 out]
        n115 = property on="Post Command Delay" class="Arr (strict)"("Number of Rows"=w156) -> ()  [unwired: 2 in, 2 out]
        n116 = property on="Device" class="RadioBtnsControl (strict)"("DisabledEnum"=w131) -> ()  [unwired: 2 in, 2 out]
        n117 = property on="Start RFFE Cycle" class="Bool"("DisabledEnum"=w140) -> ()  [unwired: 2 in, 2 out]
        n118 = property on="I2C Init" class="Bool"("DisabledEnum"=w139) -> ()  [unwired: 2 in, 2 out]
        n119 = property on="Read I2C" class="Bool"("DisabledEnum"=w139) -> ()  [unwired: 2 in, 2 out]
        n120 = property on="Write I2C" class="Bool"("DisabledEnum"=w139) -> ()  [unwired: 2 in, 2 out]
        n121 = property on="Exit" class="Bool"("DisabledEnum"=w139) -> ()  [unwired: 2 in, 2 out]
        n122 = property on="Monitor" class="Bool (strict)"("DisabledEnum"=w139) -> ()  [unwired: 2 in, 2 out]
        n123 = property on="DUT" class="Enum (strict)"("DisabledEnum"=w137) -> ()  [unwired: 2 in, 2 out]
        n124 = property on="Mode" class="RadioBtnsControl (strict)"("DisabledEnum"=w137) -> ()  [unwired: 2 in, 2 out]
        n125 = property on="Write DUT" class="Bool"("DisabledEnum"=w142) -> ()  [unwired: 2 in, 2 out]
        n126 = property on="Enable DUT" class="Bool"("DisabledEnum"=w142) -> ()  [unwired: 2 in, 2 out]
        n127 = property on="Disable DUT" class="Bool"("DisabledEnum"=w142) -> ()  [unwired: 2 in, 2 out]
        n128 = call "ACT LG Activity Log Core.vi"("Log Line"="Update", "Error In (no error)"=w159) -> ("Error Out"=w157:errorcluster)  [unwired: 12 in, 1 out]
        "Busy" <- FALSE ("Busy")
        "Status" <- "" ("Status")
      }
    }
    n129 = call <vilib>:"Simple Error Handler.vi"("error in (no error)"=w118) -> ("error out"=w128:errorcluster)  [unwired: 4 in, 4 out]
  }
  n130 = flat-sequence "Shutdown" {
    tunnel: w10 -> [w392]
    tunnel: w9 -> [w391]
    tunnel: w8 -> [_]
    tunnel: w7 -> [_]
    frame #0 {
      n131 = Release Queue(queue=w392, error in (no error)=w391) -> (error out=w390:errorcluster)  [unwired: 1 in, 2 out]
      n132 = call "WSVCAP SHL Host TL Close.vi"("error in"=w390) -> ("error out"=w389:errorcluster)  [unwired: 14 in]
      n133 = call <vilib>:"Simple Error Handler.vi"("error in (no error)"=w389) -> ()  [unwired: 4 in, 5 out]
    }
  }
